vi "graph_luz.vi"() -> ()   [LabVIEW 2021]
uses:
  <vilib>/Analysis/1siggen.llb/Ramp Pattern by Delta.vi
  <vilib>/Analysis/NI_AALBase.lvlib
panel:
  out "Curva de temperatura":cluster{"Ramp Pattern":dbl[], u32[]}(graph)
  in  "file path (dialog if empty)":path
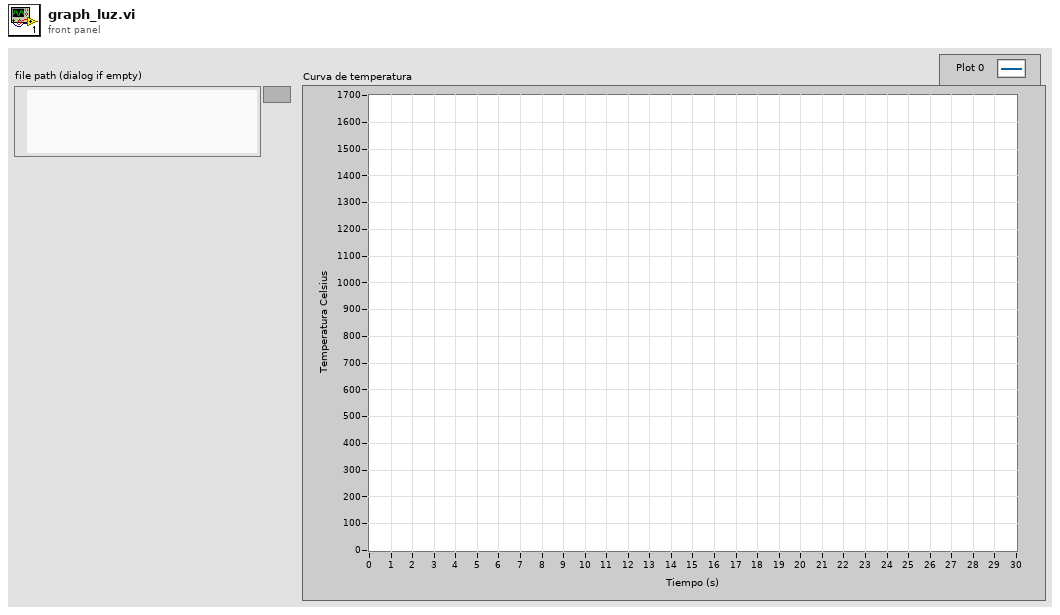
[diagram p1: front panel]
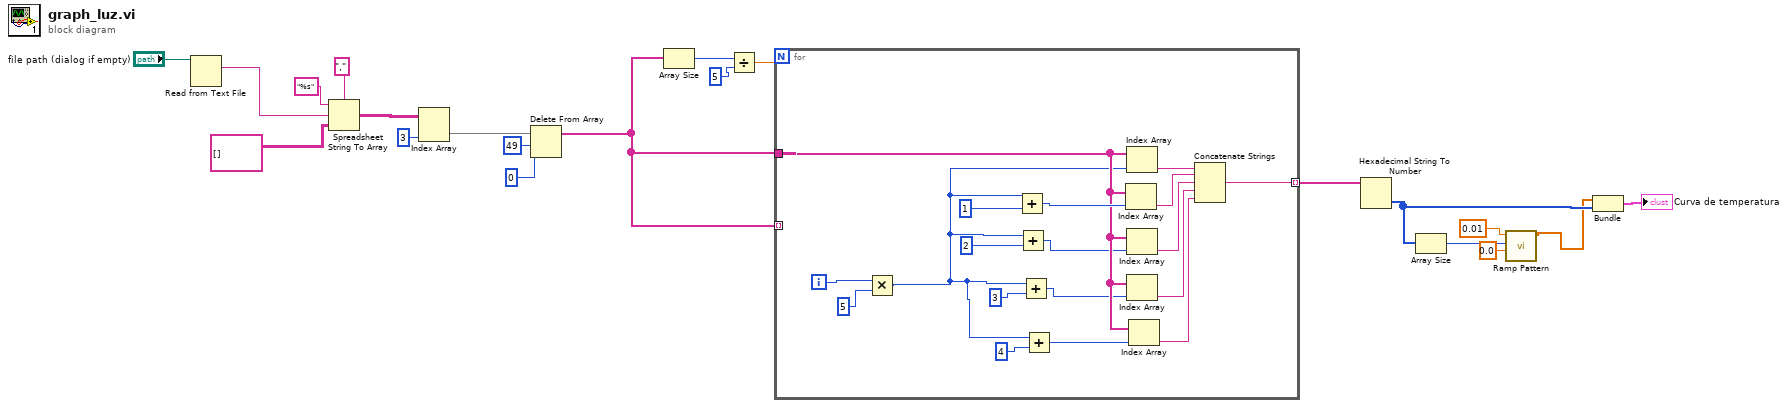
[diagram p0: block diagram]
diagram:
  n1 = Read from Text File(file (use dialog)="file path (dialog if empty)") -> (text=w19:string)  [unwired: 3 in, 3 out]
  n2 = Spreadsheet String To Array(delimiter (Tab)=",", format string="%s", spreadsheet string=w19, array type (2D Dbl)=string[][] [] ("Array")) -> (array=w16:string[][])
  n3 = Index Array(array=w16, index (col)=3 ("disabled index (col)")) -> (element=w14:string[])  [unwired: 1 in]
  n4 = Delete From Array(array=w14, length=49, index=0) -> (array with subset deleted=w11:string[])  [unwired: 1 out]
  n5 = Array Size(array=w11) -> (size(s)=w10:i32)
  n6 = Divide(x=w10, y=5) -> (x/y=w8:dbl)
  n7 = for {
    N: w8 -> [_]
    tunnel: w11 -> [_] mode=indexing
    tunnel: w11 -> [w30]
    tunnel: [w36] -> w7 mode=indexing
    i -> [w32]
    n8 = Multiply(x=w32, y=5) -> (x*y=w24:i32)
    n9 = Add(x=w24, y=1) -> (x+y=w33:i32)
    n10 = Add(x=w24, y=2) -> (x+y=w29:i32)
    n11 = Add(x=w24, y=3) -> (x+y=w28:i32)
    n12 = Add(x=w24, y=4) -> (x+y=w26:i32)
    n13 = Index Array(array=w30, index=w33) -> (element=w38:string)
    n14 = Index Array(array=w30, index=w24) -> (element=w39:string)
    n15 = Index Array(array=w30, index=w29) -> (element=w37:string)
    n16 = Index Array(array=w30, index=w28) -> (element=w23:string)
    n17 = Index Array(array=w30, index=w26) -> (element=w22:string)
    n18 = Concatenate Strings(w39, w38, w37, w23, w22) -> (w36:string)
  }
  n19 = Hexadecimal String To Number(string=w7) -> (number=w3:u32[])  [unwired: 2 in, 1 out]
  n20 = Array Size(array=w3) -> (size(s)=w6:i32)
  n21 = call-poly <vilib>:"Ramp Pattern.vi"("start"=0.0, "end"=w6, "delta"=0.01) -> ("Ramp Pattern"=w2:dbl[])  [unwired: 6 in, 2 out]
  n22 = Bundle("Ramp Pattern"=w2, w3) -> (→"Curva de temperatura":cluster{"Ramp Pattern":dbl[], u32[]})  [unwired: 1 in]
